vi "TimerManagerGV.vi"(7 "Command":enum16{"Get Time Elapsed", "Start Timer"}(ring), 9 "Hard Limit (s)":u32=40, 10 "Time to Wait (s)":u32) -> (2 "Timer Expired?":bool, 3 "Timer Value(s)":u32)   [LabVIEW 2017]
panel:
  # "default - 40 Secs"
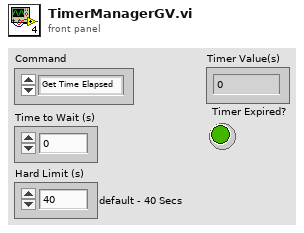
[diagram p1: front panel]
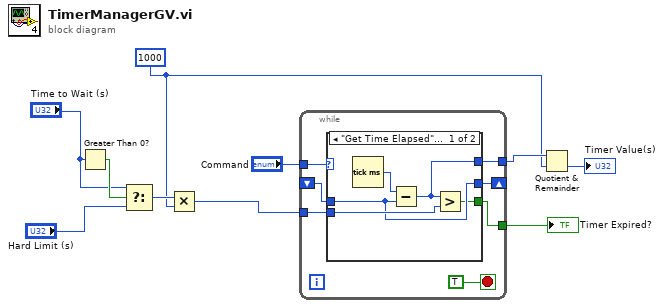
[diagram p0: block diagram]
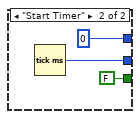
[diagram p2: hidden frame]
diagram:
  w2 = u32 1000 ("y")
  n1 = Greater Than 0?(x="Time to Wait (s)") -> (x > 0?=w8:bool)
  n2 = Select(t="Time to Wait (s)", s=w8, f="Hard Limit (s)") -> (s? t:f=w6:u32)
  n3 = Multiply(x=w6, y=w2) -> (x*y=w5:u32)
  n4 = while {
    tunnel: "Command" -> [w17]
    shift-right: [w13] -> _
    shift-left: _ -> [w15]
    tunnel: w5 -> [w14]
    tunnel: [w12] -> w3
    tunnel: [w11] -> w9
    stop <- TRUE stop-if-true
    n5 = case shown="\"Get Time Elapsed\", Default" w17 {
      tunnel: [w21 w25] -> w13
      tunnel: w15 -> [w21 _]
      tunnel: w14 -> [w22 _]
      tunnel: [w18 u32 0 ("millisecond timer value")] -> w12
      tunnel: [w19 FALSE] -> w11
      frame "Get Time Elapsed", Default {
        n6 = Tick Count (ms)() -> (millisecond timer value=w20:u32)
        n7 = Subtract(x=w20, y=w21) -> (x-y=w18:u32)
        n8 = Greater?(x=w18, y=w22) -> (0:w19:bool)
      }
      frame "Start Timer" {
        n9 = Tick Count (ms)() -> (millisecond timer value=w25:u32)
      }
    }
  }
  "Timer Expired?" <- w9
  n10 = Quotient & Remainder(x=w3, y=w2) -> (floor(x/y)=→"Timer Value(s)":u32)  [unwired: 1 out]
